vi "Find Range Check Result by Listbox Value.vi"(3 "error in (no error)":errorcluster, 4 "reference":refnum<vi>, 5 "Range Check Results in":T2(array[cluster])=[{"name"="D:OUTTMP", "value"=17.051272696256788, "range state"=0}]) -> (0 "error out":errorcluster, 1 "Found?":bool, 2 "Range Check Result out":T1)   [LabVIEW 2013, in "ACNET Monitor.lvlib"]
uses:
  ACNET Monitor.lvlib
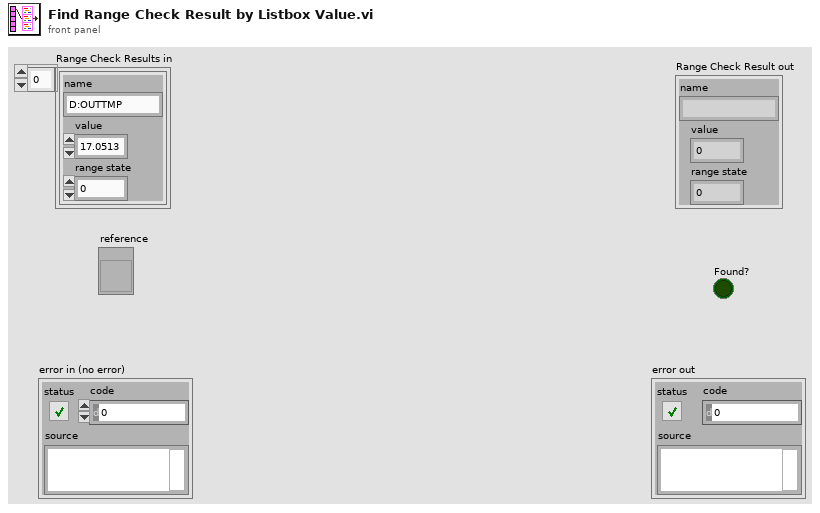
[diagram p1: front panel]
types:
  T1 = cluster{"name":string, "value":dbl, "range state":i8}
  T2 = cluster{"name":string, "value":dbl, "range state":i8}[]
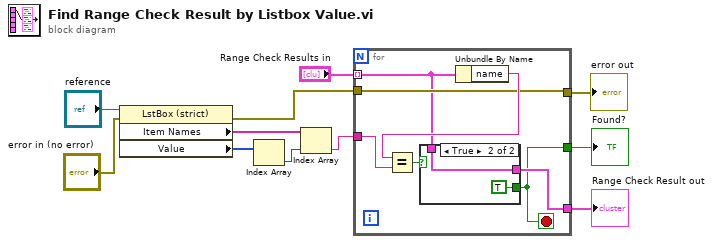
[diagram p0: block diagram]
diagram:
  n1 = property on="Property Node" class="LstBox (strict)"(reference="reference", error in="error in (no error)") -> (error out=w4:errorcluster, "Item Names"=w9:string[], "Value"=w7:i32[])  [unwired: 1 out]
  n2 = Index Array(array=w7) -> (element=w10:i32)  [unwired: 1 in]
  n3 = Index Array(array=w9, index=w10) -> (element=w11:string)
  n4 = for {
    tunnel: "Range Check Results in" -> [w12] mode=indexing
    tunnel: w4 -> [w13]
    tunnel: w11 -> [w17]
    tunnel: [w13] -> w5
    tunnel: [w15] -> w2
    tunnel: [w14] -> w1
    stop <- w14 stop-if-true
    n5 = Unbundle By Name(w12) -> ("name"=w18:string)
    n6 = Equal?(x=w18, y=w17) -> (x = y?=w16:bool)
    n7 = case shown="True" w16 {
      tunnel: [_ TRUE] -> w14
      tunnel: w12 -> [_ w19]
      tunnel: [_ w19] -> w15
      frame False {
      }
      frame True {
      }
    }
  }
  "error out" <- w5
  "Range Check Result out" <- w2
  "Found?" <- w1
